vi "Teleop.vi"(10 "Match Info":T1={"Autonomous Elapsed Seconds"=0.0, "TeleOp Elapsed Seconds"=0.0, "Disabled Elapsed Seconds"=0.0, "Visited Autonomous"=FALSE, "Visited TeleOp"=FALSE, "Visited Disabled"=FALSE, "Autonomous Settings"={"Autonomous Style"=enum."Independent", "VI Refnum"=refnum}}, 11 "Call Context":T2) -> ()   [LabVIEW 2017]
doc: "This VI is called for each TeleOp packet received from the DS where the robot is not disabled. It is often used to read from the joysticks and update I/O or to update setpoints for timed control loops. It should complete and return within 20 milliseconds or it may miss DS packets."
uses:
  <vilib>/Rock Robotics/WPI/DriverStation/WPI_DriverStationDerivedRobotMode.ctl
  <vilib>/Rock Robotics/WPI/DriverStation/WPI_DriverStationMatch Info.ctl
  <vilib>/Rock Robotics/WPI/Solenoid/WPI_SolenoidValue.ctl
  <vilib>/Rock Robotics/WPI/Utilities/WPI_GetSetVariantRefNum.vi
  <vilib>/Rock Robotics/Network Tables/NT Write Boolean Array.vi
  <vilib>/Rock Robotics/Network Tables/NT Write Numeric Array.vi
  <vilib>/Rock Robotics/Network Tables/NT Read Boolean.vi
  <vilib>/Rock Robotics/Network Tables/NT Read Number.vi
  Robot Global Data.vi
  <vilib>/Rock Robotics/Network Tables/NT Write Boolean.vi
  <vilib>/Rock Robotics/WPI/Solenoid/WPI_SolenoidSetEnum.vi
panel:
  out "Sample Slider 0":dbl(slide) scale=0.0..5.0
  out "Sample Boolean 1":bool
  out "Sample Boolean 0":bool
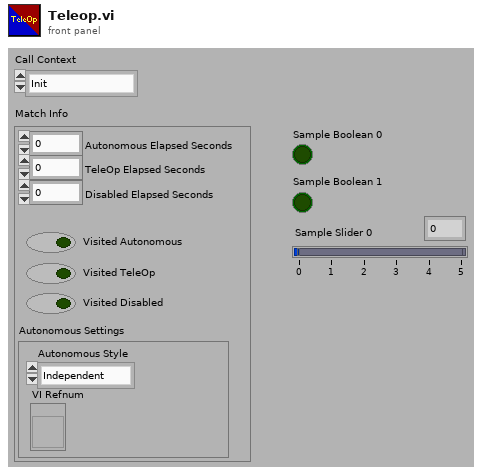
[diagram p1: front panel]
types:
  T1 = typedef "WPI_DriverStationMatch Info.ctl" = cluster{"Autonomous Elapsed Seconds":dbl, "TeleOp Elapsed Seconds":dbl, "Disabled Elapsed Seconds":dbl, "Visited Autonomous":bool, "Visited TeleOp":bool, "Visited Disabled":bool, "Autonomous Settings":cluster{"Autonomous Style":enum16{"Iterative", "Independent"}, "VI Refnum":refnum<vi>}}
  T2 = typedef "WPI_DriverStationDerivedRobotMode.ctl" = enum16{"Init", "Execute", "Stop"}
  T3 = typedef "WPI_SolenoidValue.ctl" = enum16{"Off", "On", "Forward", "Reverse"}
  T4 = enum16{"Linear", "Square  Root", "Square", "n^x"}
  T5 = typedef "WPI_JoystickDevRef.ctl" = cluster{"Device":T6}
  T6 = typedef "WPI_JoystickDeviceEnum.ctl" = enum16{"USB 0", "USB 1", "USB 2", "USB 3", "USB 4", "USB 5"}
  T7 = typedef "WPI_MotorControlDeviceRef.ctl" = cluster{"DeviceStatus":errorcluster, "Type":T8, "PWM":cluster{"PWM Channel":T9, "DeadBand":T10}, "CAN":cluster{"Device Number":u8, "SetOutput VI Ref":variant, "GetOutput VI Ref":variant, "Enable VI Ref":variant, "Disable VI Ref":variant, "Data":variant}, "Invert":bool, "DIO PWM":cluster{"PWM \"Enable\" Channel":T9, "DIOChannel":T11, "PWM Rate":dbl}}
  T8 = typedef "WPI_MotorControlType.ctl" = enum16{"PWM", "CAN", "DIO PWM"}
  T9 = typedef "FPGA_DIOPWMChannel.ctl" = enum8{"PWM 0", "PWM 1", "PWM 2", "PWM 3", "PWM 4", "PWM 5", "PWM 6", "PWM 7", "PWM 8", "PWM 9", "PWM MXP 0", "PWM MXP 1", "PWM MXP 2", "PWM MXP 3", "PWM MXP 4", "PWM MXP 5", "PWM MXP 6", "PWM MXP 7", "PWM MXP 8", "PWM MXP 9", "Invalid"}
  T10 = typedef "WPI_PWMDeadband.ctl" = cluster{"Name":string, "maxPositivePwm":i32, "minPositivePwm":i32, "centerPwm":i32, "maxNegativePwm":i32, "minNegativePwm":i32, "angularRange":u16}
  T11 = typedef "FPGA_DIOChannel.ctl" = enum8{"DIO 0", "DIO 1", "DIO 2", "DIO 3", "DIO 4", "DIO 5", "DIO 6", "DIO 7", "DIO 8", "DIO 9", "DIO MXP 0", "DIO MXP 1", "DIO MXP 2", "DIO MXP 3", "DIO MXP 4", "DIO MXP 5", "DIO MXP 6", "DIO MXP 7", "DIO MXP 8", "DIO MXP 9", "DIO MXP 10", "DIO MXP 11", "DIO MXP 12", "DIO MXP 13", "DIO MXP 14", "DIO MXP 15", "SPI Port CS1", "SPI Port CS2", "SPI Port CS3", "SPI Port MISO", "SPI Port MOSI", "Invalid"}
  T12 = typedef "WPI_SolenoidDevRef.ctl" = cluster{"DevStatus":errorcluster, "Pneumatics Control Module":u8, "Forward Solenoid Channel":T13, "Reverse Solenoid Channel":T13}
  T13 = typedef "WPI_SolenoidChannel.ctl" = enum8{"Solenoid 0", "Solenoid 1", "Solenoid 2", "Solenoid 3", "Solenoid 4", "Solenoid 5", "Solenoid 6", "Solenoid 7", "Invalid"}
  T14 = cluster{"X":dbl, "Y":dbl, "Angle":dbl, "Magnitude":dbl}
  T15 = typedef "WPI_RobotDriveDevRef.ctl" = cluster{"DevStatus":errorcluster, "Motors[]":T7[], "Square Inputs":bool, "Max Output":dbl}
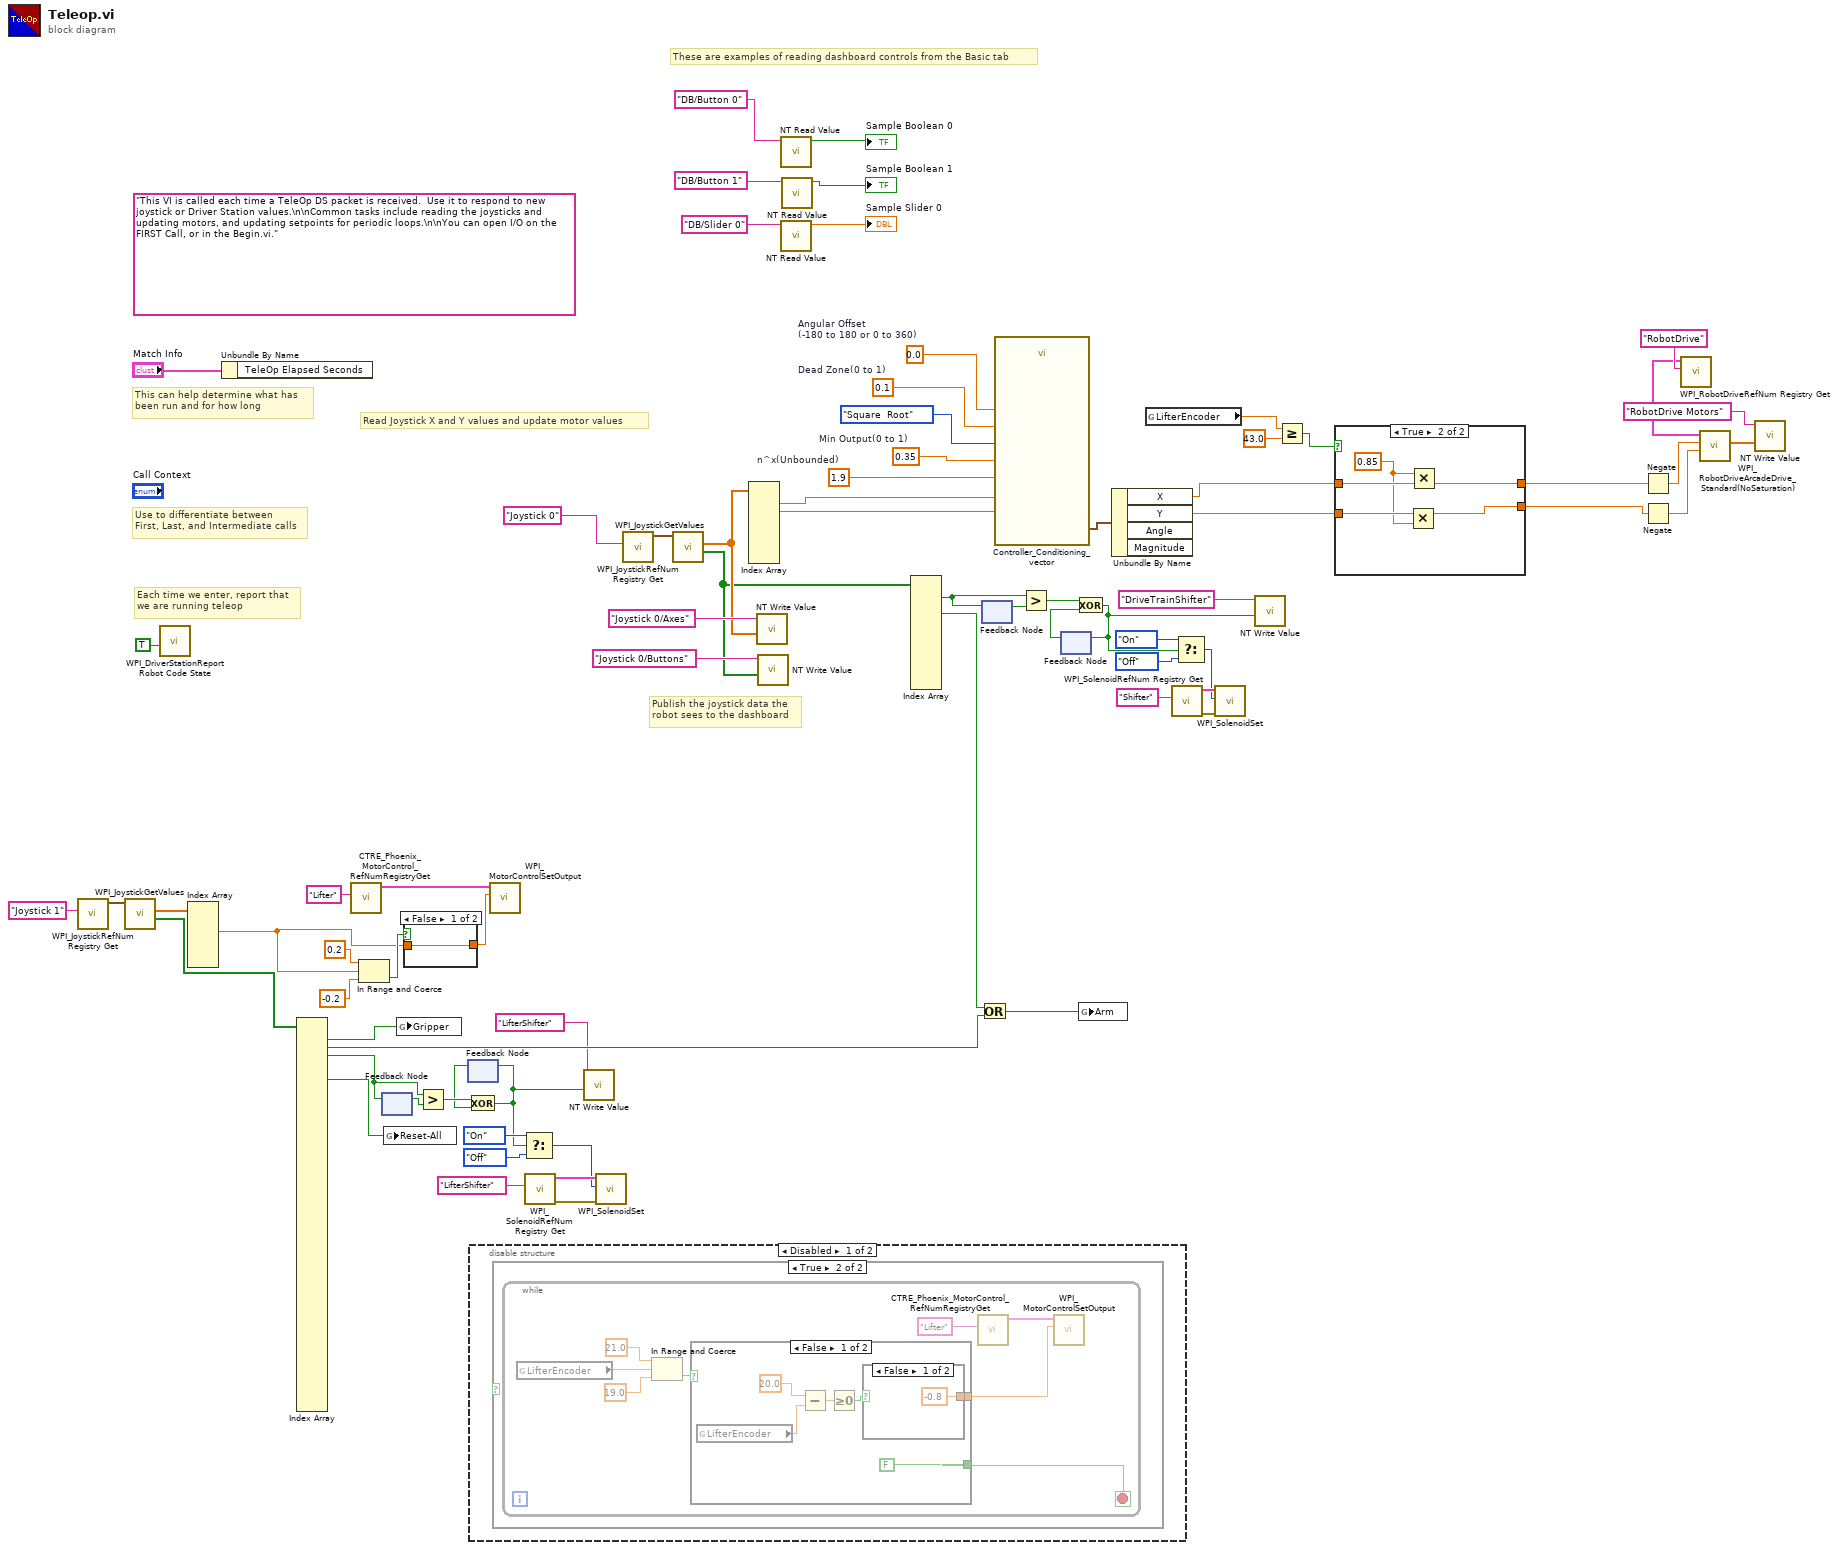
[diagram p0: block diagram]
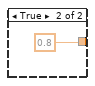
[diagram p4: hidden frame]
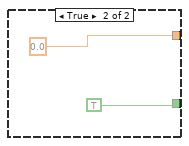
[diagram p5: hidden frame]
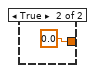
[diagram p7: hidden frame]
diagram:
  w21 = 1.9  # n^x(Unbounded)
  w22 = 0.35  # Min Output(0 to 1)
  w24 = 0.1  # Dead Zone(0 to 1)
  w25 = 0.0  # Angular Offset (-180 to 180 or 0 to 360)
  (unwired) "This VI is called each time a TeleOp DS packet is received.  Use it to respond to new joystick or Driver Station values.\n\nCommon tasks include reading the joysticks and updating motors, and updating setpoints for periodic loops.\n\nYou can open I/O on the FIRST Call, or in the Begin.vi."
  # "These are examples of reading dashboard controls from the Basic tab"
  # "Publish the joystick data the\nrobot sees to the dashboard"
  # "Each time we enter, report that\nwe are running teleop"
  # "Use to differentiate between\nFirst, Last, and Intermediate calls"
  # "This can help determine what has\nbeen run and for how long"
  # "Read Joystick X and Y values and update motor values"
  n1 = call <vilib>:"WPI_JoystickRefNum Registry Get.vi"("refnum name"="Joystick 1") -> ("JoystickDevRef"=w57:T5)  [unwired: 1 in, 9 out]
  n2 = call <vilib>:"WPI_JoystickGetValues.vi"("JoystickDevRef"=w57) -> ("Buttons"=w53:bool[], "Axes"=w56:dbl[])  [unwired: 6 in, 3 out]
  n3 = call <vilib>:"WPI_DriverStationReport Robot Code State.vi"("TeleOp"=TRUE ("Autonomous")) -> ()  [unwired: 10 in, 1 out]
  n4 = Index Array(array=w56) -> (element #2=w38:dbl)  [unwired: 6 in, 5 out]
  n5 = Unbundle By Name("Match Info") -> ()  [unwired: 1 out]
  n6 = Index Array(array=w53) -> (element #1=w37:bool, element #2=w35:bool, element #3=w34:bool, element #6=w12:bool)  [unwired: 47 in, 43 out]
  n7 = call <vilib>:"CTRE_Phoenix_MotorControl_RefNumRegistryGet.vi"("refnum name"="Lifter") -> ("PhoenixMotorControlDevRef"=w55:T7)  [unwired: 9 in, 1 out]
  n8 = In Range and Coerce(upper limit=0.2, x=w38, lower limit=-0.2) -> (In Range?=w40:bool)  [unwired: 1 out]
  n9 = feedback #1() -> (w49:bool)  [unwired: 1 in]
  n10 = feedback-in #1(w34) -> ()
  n11 = global write "Robot Global Data.vi" "Reset-All"(w12) -> ()
  n12 = global write "Robot Global Data.vi" "Gripper"(w37) -> ()
  n13 = case shown="False" w40 {
    tunnel: [w76 0.0 ("Output")] -> w39
    tunnel: w38 -> [w76 _]
    frame False {
    }
    frame True {
    }
  }
  n14 = Greater?(x=w34, y=w49) -> (0:w48:bool)
  n15 = feedback #2() -> (w47:bool)  [unwired: 1 in]
  n16 = Exclusive Or(1:w47, 2:w48) -> (0:w9:bool)
  n17 = feedback-in #2(w9) -> ()
  n18 = disable-structure shown="Disabled" {
    frame Disabled {
      n19 = case shown="True" {
        selector: _ -> [_ _]
        frame False {
          # "sohcahtoa"
        }
        frame True {
          n20 = while {
            stop <- w78 stop-if-true
            n21 = global read "Robot Global Data.vi" "LifterEncoder"() -> (w85:dbl)
            n22 = In Range and Coerce(upper limit=21.0, x=w85, lower limit=19.0) -> (In Range?=w82:bool)  [unwired: 1 out]
            n23 = case shown="False" w82 {
              tunnel: [w90 0.0] -> w79
              tunnel: [FALSE TRUE] -> w78
              frame False {
                n24 = global read "Robot Global Data.vi" "LifterEncoder"() -> (w89:dbl)
                n25 = Subtract(x=20.0, y=w89) -> (x-y=w87:dbl)
                n26 = Greater Or Equal To 0?(x=w87) -> (x >= 0?=w86:bool)
                n27 = case shown="False" w86 {
                  tunnel: [-0.8 0.8] -> w90
                  frame False {
                  }
                  frame True {
                  }
                }
              }
              frame True {
              }
            }
            n28 = call <vilib>:"CTRE_Phoenix_MotorControl_RefNumRegistryGet.vi"("refnum name"="Lifter") -> ("PhoenixMotorControlDevRef"=w81:T7)  [unwired: 9 in, 1 out]
            n29 = call <vilib>:"WPI_MotorControlSetOutput.vi"("Output"=w79, "MotorControlDevRef"=w81) -> ()  [unwired: 7 in, 3 out]
          }
        }
      }
    }
    frame Enabled {
    }
  }
  n30 = call <vilib>:"WPI_MotorControlSetOutput.vi"("Output"=w39, "MotorControlDevRef"=w55) -> ()  [unwired: 7 in, 3 out]
  n31 = Select(t=WPI_SolenoidValue."On" ("Value"), s=w9, f=WPI_SolenoidValue."Off" ("Value")) -> (s? t:f=w44:T3)
  n32 = call <vilib>:"WPI_SolenoidRefNum Registry Get.vi"("refnum name"="LifterShifter") -> ("error out"=w51:errorcluster, "SolenoidDevRef"=w50:T12)  [unwired: 9 in]
  n33 = call-poly <vilib>:"NT Write Value.vi"("Boolean"=w9, "Name"="LifterShifter") -> ()  [unwired: 9 in, 1 out]
  n34 = call-poly <vilib>:"WPI_SolenoidSet.vi"("error in (no error)"=w51, "Value"=w44, "SolenoidDevRef"=w50) -> ()  [unwired: 7 in, 2 out]
  n35 = call <vilib>:"WPI_JoystickRefNum Registry Get.vi"("refnum name"="Joystick 0") -> ("JoystickDevRef"=w73:T5)  [unwired: 1 in, 9 out]
  n36 = call <vilib>:"WPI_JoystickGetValues.vi"("JoystickDevRef"=w73) -> ("Buttons"=w62:bool[], "Axes"=w69:dbl[])  [unwired: 6 in, 3 out]
  n37 = Index Array(array=w69) -> (element #1=w27:dbl, element #2=w26:dbl)  [unwired: 8 in, 6 out]
  n38 = call-poly <vilib>:"NT Write Value.vi"("Numeric Array"=w69, "Name"="Joystick 0/Axes") -> ()  [unwired: 9 in, 1 out]
  n39 = call-poly <vilib>:"NT Write Value.vi"("Boolean Array"=w62, "Name"="Joystick 0/Buttons") -> ()  [unwired: 9 in, 1 out]
  n40 = call-poly <vilib>:"NT Read Value.vi"("Name"="DB/Button 0" ("refnum name")) -> ("Boolean"=→"Sample Boolean 0":bool)  [unwired: 9 in, 1 out]
  n41 = call-poly <vilib>:"NT Read Value.vi"("Name"="DB/Slider 0" ("refnum name")) -> ("Numeric"=→"Sample Slider 0":dbl)  [unwired: 9 in, 1 out]
  n42 = call-poly <vilib>:"NT Read Value.vi"("Name"="DB/Button 1" ("refnum name")) -> ("Boolean"=→"Sample Boolean 1":bool)  [unwired: 9 in, 1 out]
  n43 = Index Array(array=w62) -> (element #1=w13:bool, element #3=w43:bool)  [unwired: 12 in, 10 out]
  n44 = Or(x=w43, y=w35) -> (x .or. y?=w36:bool)
  n45 = feedback #3() -> (w15:bool)  [unwired: 1 in]
  n46 = feedback-in #3(w13) -> ()
  n47 = call "Controller_Conditioning_vector.vi"("Angular Offset\n(-180 to 180 or 0 to 360)"=w25, "Min Output(0 to 1)"=w22, "n^x(Unbounded)"=w21, "Enum"=T4."Square  Root", "Dead Zone(0 to 1)"=w24, "Y(-1 to 1)"=w26, "X(-1 to 1)"=w27) -> ("output cluster"=w20:T14)  [unwired: 4 in]
  n48 = Greater?(x=w13, y=w15) -> (0:w19:bool)
  n49 = feedback #4() -> (w18:bool)  [unwired: 1 in]
  n50 = Exclusive Or(1:w18, 2:w19) -> (0:w11:bool)
  n51 = feedback-in #4(w11) -> ()
  n52 = global write "Robot Global Data.vi" "Arm"(w36) -> ()
  n53 = Unbundle By Name(w20) -> ("X"=w4:dbl, "Y"=w6:dbl)  [unwired: 2 out]
  n54 = global read "Robot Global Data.vi" "LifterEncoder"() -> (w1:dbl)
  n55 = call <vilib>:"WPI_SolenoidRefNum Registry Get.vi"("refnum name"="Shifter") -> ("error out"=w60:errorcluster, "SolenoidDevRef"=w59:T12)  [unwired: 9 in]
  n56 = Select(t=WPI_SolenoidValue."On" ("Value"), s=w11, f=WPI_SolenoidValue."Off" ("Value")) -> (s? t:f=w14:T3)
  n57 = call-poly <vilib>:"WPI_SolenoidSet.vi"("error in (no error)"=w60, "Value"=w14, "SolenoidDevRef"=w59) -> ()  [unwired: 7 in, 2 out]
  n58 = call-poly <vilib>:"NT Write Value.vi"("Boolean"=w11, "Name"="DriveTrainShifter") -> ()  [unwired: 9 in, 1 out]
  n59 = Greater Or Equal?(x=w1, y=43.0) -> (x >= y?=w3:bool)
  n60 = case shown="True" w3 {
    tunnel: [w96 w99] -> w7
    tunnel: w6 -> [w96 w102]
    tunnel: [w97 w100] -> w5
    tunnel: w4 -> [w97 w101]
    frame False {
    }
    frame True {
      w98 = 0.85 ("x")
      n61 = Multiply(x=w102, y=w98) -> (x*y=w99:dbl)
      n62 = Multiply(x=w98, y=w101) -> (x*y=w100:dbl)
    }
  }
  n63 = Negate(x=w5) -> (-x=w29:dbl)
  n64 = Negate(x=w7) -> (-x=w28:dbl)
  n65 = call <vilib>:"WPI_RobotDriveRefNum Registry Get.vi"("refnum name"="RobotDrive") -> ("RobotDriveDevRef"=w32:T15)  [unwired: 1 in, 9 out]
  n66 = call <vilib>:"WPI_RobotDriveArcadeDrive_Standard(NoSaturation).vi"("Y axis value"=w28, "X axis value"=w29, "RobotDriveDevRef"=w32) -> ("Motor Values"=w31:dbl[])  [unwired: 1 in, 7 out]
  n67 = call-poly <vilib>:"NT Write Value.vi"("Numeric Array"=w31, "Name"="RobotDrive Motors") -> ()  [unwired: 9 in, 1 out]
